vi "Configure VI Tester.vi"(8 "error in (no error)":errorcluster, 10 "JSON String":string) -> (0 "error out":errorcluster, 3 "Run VI Tester out":refnum<class "Run VI Tester.lvclass">)   [LabVIEW 2014, in "Run VI Tester.lvclass"]
uses:
  Run VI Tester.lvclass
  Shared/Controls/VI Tester - STYP.ctl
  Classes/Job/Job.lvclass/Job.ctl
  Run VI Tester.lvclass/Run VI Tester.ctl
  Classes/Job/Job.lvclass
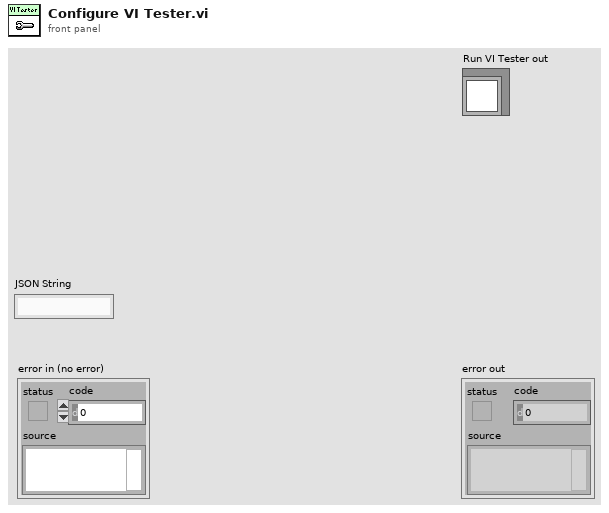
[diagram p1: front panel]
types:
  T1 = typedef "VI Tester - STYP.ctl" = cluster{"Executor_Number":string, "Workspace_Path":string, "Test Case":string}
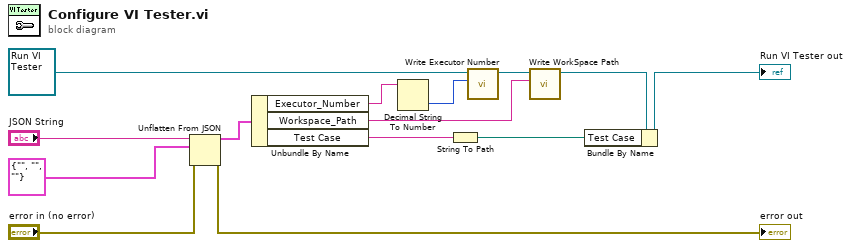
[diagram p0: block diagram]
diagram:
  n1 = Unflatten From JSON(JSON string="JSON String", type and defaults=T1 {"Executor_Number"="", "Workspace_Path"="", "Test Case"=""} ("VI Analyzer - STYP.ctl"), error in (no error)="error in (no error)") -> (value=w13:T1, error out=→"error out":errorcluster)  [unwired: 4 in]
  n2 = Unbundle By Name(w13) -> ("Executor_Number"=w12:string, "Workspace_Path"=w9:string, "Test Case"=w7:string)
  n3 = Decimal String To Number(string=w12) -> (number=w10:i32)  [unwired: 2 in, 1 out]
  n4 = String To Path(string=w7) -> (path=w6:path)
  n5 = call "Write Executor Number.vi"("Executor Number"=w10, "Job in"=refnum<class "Run VI Tester.lvclass"> refnum ("Run VI Tester in")) -> ("Job out"=w11:refnum<class "Run VI Tester.lvclass">)  [unwired: 8 in, 1 out]
  n6 = call "Write WorkSpace Path.vi"("WorkSpace Path"=w9, "Job in"=w11) -> ("Job out"=w8:refnum<class "Run VI Tester.lvclass">)  [unwired: 8 in, 1 out]
  n7 = Bundle By Name(cluster=w8, "Test Case"=w6) -> (→"Run VI Tester out":refnum<class "Run VI Tester.lvclass">)
